vi "断电保存全局变量.vi"() -> ()   [LabVIEW 2016, in "环境动力监测库.lvlib"]
uses:
  <vilib>/Plasmionique/MB Master/MB_Master/MB_Master.lvclass
panel:
  in  "选项卡控件":T1(tab)
  in  "空调全局":T2={"型号选择"=enum."黑盾", "MB session in"=refnum, "英维克空调寄存器"=[], "通讯状态"=TRUE, "PORT"="502", "IP"="192.168.1.207", "Slave ID "=1, "Serial Config"={"baud rate (bps)"=9600, "stop bits"=10, "parity"=0, "flow control"=0, "timeout"=1000, "retries"=1}, "VISA Resource"="COM1", "MB通信方式选择"=enum."串口"} {"Serial Config"."stop bits" items=["1.0"=10, "1.5"=15, "2.0"=20]; "Serial Config"."flow control" items=["None", "XON/XOFF", "RTS/CTS", "XON/XOFF & RTS/CTS", "DTR/DSR", "XON/XOFF & DTR/DSR"]; "Serial Config"."parity" items=["None", "Odd", "Even", "Mark", "Space"]}
  in  "UPS全局":T3={"VISA resource name"="", "Serial Config"={"baud rate (9600)"=2400, "stop bits (10: 1 bit)"=10, "parity (0:none)"=enum."None", "data bits (8)"=8, "timeout (10sec)"=10000}, "型号选择"=enum."山特UPSC1~3", "HW-UPS-2000 MB session"=refnum, "连接方式"=enum."串口", "IP"="", "Port"=""} {"Serial Config"."data bits (8)" min=5 max=8 step=1; "Serial Config"."stop bits (10: 1 bit)" items=["1.0"=10, "1.5"=15, "2.0"=20]}
  out "累计用电量KW·h":dbl
  in  "MPPT-12 Serial":refnum<visa-resource-name>
  in  "MPPT-24 Serial":refnum<visa-resource-name>
  in  "MPPT12电量告警":dbl
  in  "MPPT24电量告警":dbl
  in  "MPPT-12Serial Config":T4={"baud rate (bps)"=115200, "stop bits"=10, "parity"=0, "flow control"=0, "timeout"=1000, "retries"=1} {"stop bits" items=["1.0"=10, "1.5"=15, "2.0"=20]; "parity" items=["None", "Odd", "Even", "Mark", "Space"]; "flow control" items=["None", "XON/XOFF", "RTS/CTS", "XON/XOFF & RTS/CTS", "DTR/DSR", "XON/XOFF & DTR/DSR"]}
  in  "MPPT-24Serial Config":T4={"baud rate (bps)"=115200, "stop bits"=10, "parity"=0, "flow control"=0, "timeout"=1000, "retries"=1} {"stop bits" items=["1.0"=10, "1.5"=15, "2.0"=20]; "parity" items=["None", "Odd", "Even", "Mark", "Space"]; "flow control" items=["None", "XON/XOFF", "RTS/CTS", "XON/XOFF & RTS/CTS", "DTR/DSR", "XON/XOFF & DTR/DSR"]}
  in  "MPPT-12站号":u64
  in  "MPPT-24站号":u64
  in  "纬度":dbl
  in  "经度":dbl
  in  "BD连接方式":enum16{"串口", "TCP"}(ring)
  in  "BDPort:":string
  in  "BDIP address:":string
  in  "GPS连接方式":enum16{"串口", "TCP"}(ring)
  in  "GPSPort:":string
  in  "GPSIP address:":string
  in  "手动设置定位":bool caption="定位自动获取OFF/手动设置ON"
  in  "收方地址":string="968314"
  in  "GPS移位报警设定值":dbl=1000.0
  in  "BD移位报警设定值":dbl=1000.0
  in  "GPS波特率":u32(ring)=115200 items=["4800"=4800, "9600"=9600, "38400"=38400, "19200"=19200, "115200"=115200]
  in  "GPS VISA资源名称":refnum<visa-resource-name>
  in  "BD波特率":u32(ring)=115200 items=["4800"=4800, "9600"=9600, "38400"=38400, "19200"=19200, "115200"=115200]
  in  "BDVISA资源名称":refnum<visa-resource-name>
  in  "室温上限告警点":dbl
  in  "室温下限告警点":dbl
  in  "湿度上限告警点":dbl
  in  "湿度下限告警点":dbl
  in  "高温告警开关":bool
  in  "冰箱参数":cluster{"功能启用":bool, "开启时间":u16, "关闭时间":u16}={"功能启用"=FALSE, "开启时间"=6, "关闭时间"=20} {"关闭时间" items=["00H", "01H", "02H", "03H", "04H", "05H", "06H", "07H", "08H", "09H", "10H", "11H", "12H", "13H", "14H", "15H", "16H", "17H", "18H", "19H", "20H", "21H", "22H", "23H", "关闭"]; "开启时间" items=["00H", "01H", "02H", "03H", "04H", "05H", "06H", "07H", "08H", "09H", "10H", "11H", "12H", "13H", "14H", "15H", "16H", "17H", "18H", "19H", "20H", "21H", "22H", "23H", "关闭"]}
  in  "排气扇参数":T5={"功能启用"=FALSE, "排气扇开启温度"=50.0, "排气扇关闭温度"=40.0}
  out "AD当前转换值":T6 {"AD7" format="%.2f"; "AD6" format="%.2f"; "AD5" format="%.2f"; "AD4" format="%.2f"; "AD3" format="%.2f"; "AD2" format="%.2f"; "AD1" format="%.2f"; "AD0" format="%.2f"}
  out "AD当前原始值":T7 {"AD7" format="%.2f"; "AD6" format="%.2f"; "AD5" format="%.2f"; "AD4" format="%.2f"; "AD3" format="%.2f"; "AD1" format="%.2f"; "AD1" format="%.2f"; "AD0" format="%.2f"}
  in  "AD线性关系":T8(array[cluster])=[{"X0"=1638.0, "X1"=8191.0, "Y0"=-40.0, "Y1"=100.0}, {"X0"=1638.0, "X1"=8191.0, "Y0"=0.0, "Y1"=100.0}, {"X0"=1638.0, "X1"=8191.0, "Y0"=0.0, "Y1"=1.0}, {"X0"=0.0, "X1"=8191.0, "Y0"=0.0, "Y1"=8191.0}, {"X0"=0.0, "X1"=8191.0, "Y0"=0.0, "Y1"=8191.0}, {"X0"=0.0, "X1"=8191.0, "Y0"=0.0, "Y1"=8191.0}, {"X0"=0.0, "X1"=8191.0, "Y0"=0.0, "Y1"=8191.0}, {"X0"=0.0, "X1"=8191.0, "Y0"=0.0, "Y1"=8191.0}]
  out "配置ItemNames":string[][](array[string])
  out "监测设备配置":T9
  in  "IO监测配置输入":T10
  in  "卡号信息":string[][](array[string])
  in  "红外入侵信号持续时间":u32=1 format="%.0fS"
  in  "漏水信号持续时间":u32=1 format="%.0fS"
  in  "门禁信号持续时间":u32=1 format="%.0fS"
  in  "烟雾信号持续时间":u32=1 format="%.0fS"
  in  "用水量信号持续时间":u32=1 format="%.0fS"
  in  "振动信号持续时间":u32=1 format="%.0fS"
  in  "废液信号持续时间":u32=1 format="%.0fS"
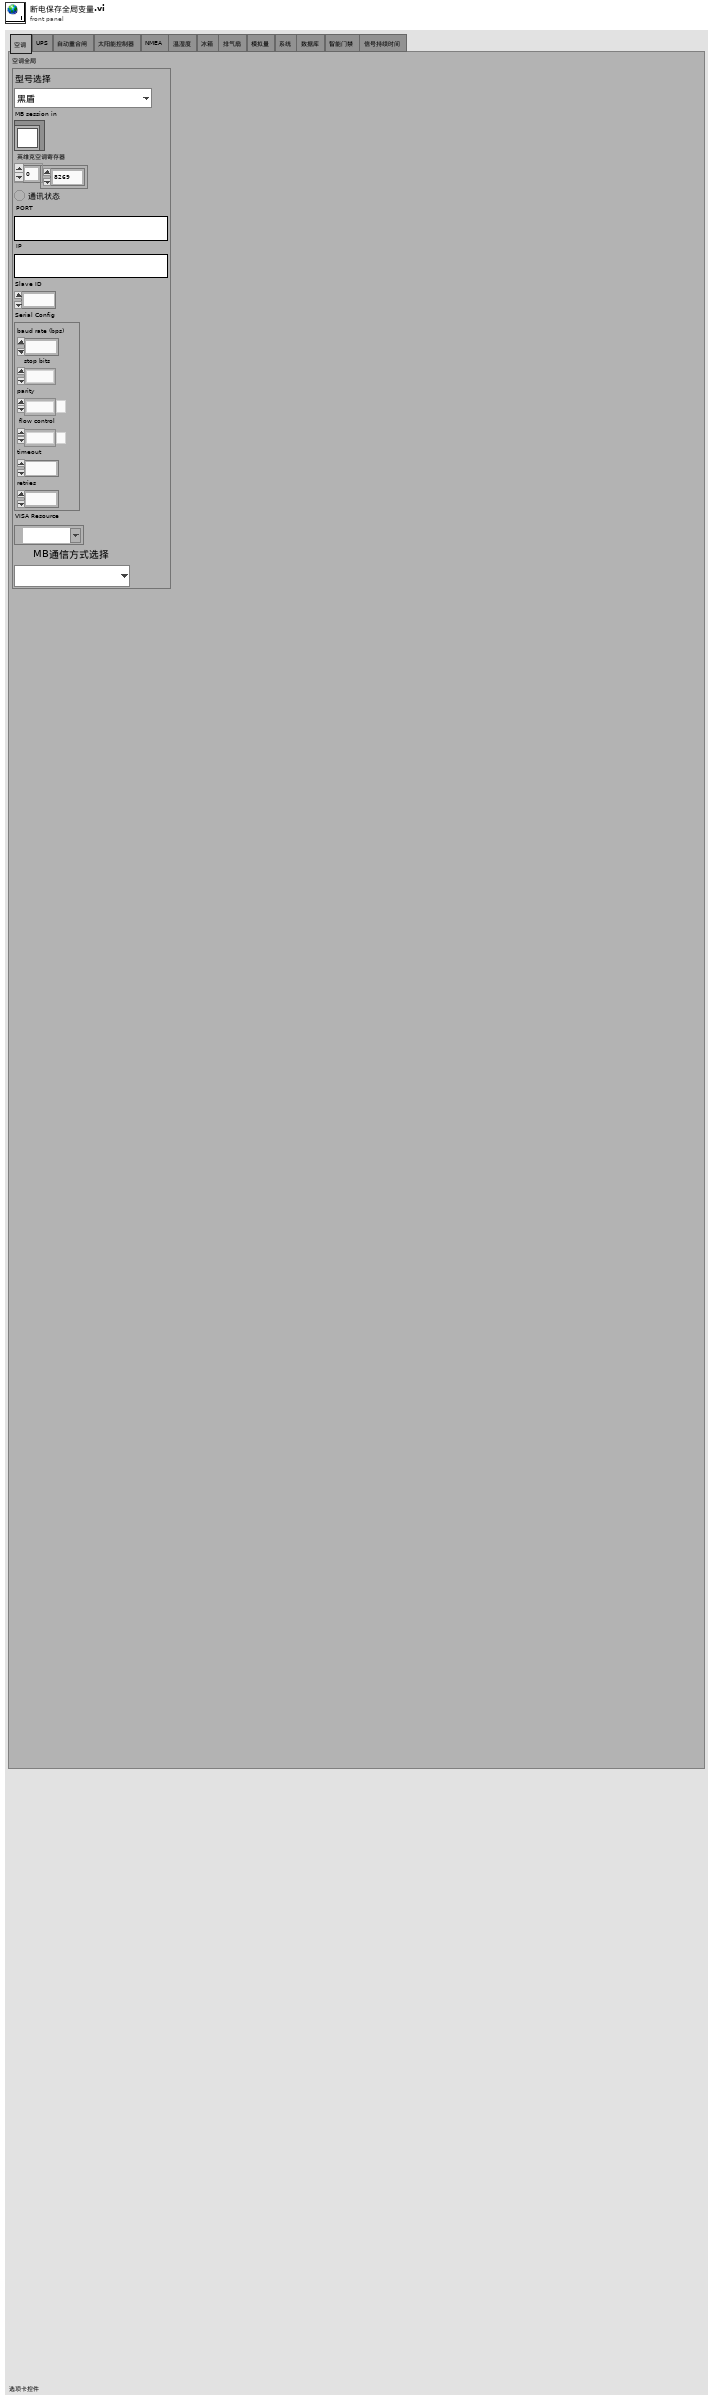
[diagram p1: front panel]
types:
  T1 = enum32{"空调", "UPS", "自动重合闸", "太阳能控制器", "NMEA", "温湿度", "冰箱", "排气扇", "模拟量", "系统", "数据库", "智能门禁", "信号持续时间"}
  T2 = cluster{"型号选择":enum16{"黑盾", "英维克", "仁科测控RS-KTC-N01"}, "MB session in":refnum<class "MB_Master.lvclass">, "英维克空调寄存器":u16[], "通讯状态":bool, "PORT":string, "IP":string, "Slave ID ":u8, "Serial Config":cluster{"baud rate (bps)":u32, "stop bits":u16, "parity":u16, "flow control":u16, "timeout":u32, "retries":i32}, "VISA Resource":refnum<visa-resource-name>, "MB通信方式选择":enum16{"串口", "TCP"}}
  T3 = cluster{"VISA resource name":refnum<visa-resource-name>, "Serial Config":cluster{"baud rate (9600)":u32, "stop bits (10: 1 bit)":u16, "parity (0:none)":enum16{"None", "Odd", "Even", "Mark", "Space"}, "data bits (8)":u16, "timeout (10sec)":u32}, "型号选择":enum16{"山特UPSC1~3", "山特UPSC6~20", "华为UPS2000-G-(1-3KVA)"}, "HW-UPS-2000 MB session":refnum<class "MB_Master.lvclass">, "连接方式":enum16{"串口", "TCP"}, "IP":string, "Port":string}
  T4 = cluster{"baud rate (bps)":u32, "stop bits":u16, "parity":u16, "flow control":u16, "timeout":u32, "retries":i32}
  T5 = cluster{"功能启用":bool, "排气扇开启温度":dbl, "排气扇关闭温度":dbl}
  T6 = cluster{"AD0":dbl, "AD1":dbl, "AD2":dbl, "AD3":dbl, "AD4":dbl, "AD5":dbl, "AD6":dbl, "AD7":dbl}
  T7 = cluster{"AD0":dbl, "AD1":dbl, "AD1":dbl, "AD3":dbl, "AD4":dbl, "AD5":dbl, "AD6":dbl, "AD7":dbl}
  T8 = cluster{"X0":dbl, "X1":dbl, "Y0":dbl, "Y1":dbl}[]
  T9 = cluster{"市电监测":bool, "用水量监测":bool, "烟雾监测":bool, "温度湿度":bool, "振动监测":bool, "红外入侵监测":bool, "漏水监测":bool, "门禁开关监测":bool, "门禁开关监测2":bool, "视频监测":bool, "UPS监测":bool, "空调监测":bool, "冰箱监测":bool, "排气扇监测":bool, "蓄电池监测":bool, "蓄电池监测2":bool, "GPS监测":bool, "北斗监测":bool, "气象监测":bool, "智能门禁监测":bool, "废液监测":bool, "废液监测2":bool}
  T10 = cluster{"漏水监测配置":cluster{"监测项描述:输出":string, "端口:":enum16{"AI0", "AI1", "AI2", "AI3", "AI4", "DI0", "DI1", "DI2", "DI3", "DI4", "DI5", "DI6", "DI7", "DO0", "DO1", "DO2", "DO3", "DO4", "DO5", "DO6", "DO7", "X0", "X1", "X2", "X3", "X4", "X5", "X6", "X7", "X8", "X9", "X10", "X11", "X12", "X13", "X14", "X15", "X16", "X17", "X18", "X19", "X20", "X21", "X22", "X23"}, "告警参数:":enum32{"禁用告警", "闭合告警", "断开告警"}, "传感器型号:":enum16{"PLC", "ZLAN", "ART"}, "声光告警启用":bool}, "门禁开关监测配置":cluster{"监测项描述:输出":string, "端口:":enum16{"AI0", "AI1", "AI2", "AI3", "AI4", "DI0", "DI1", "DI2", "DI3", "DI4", "DI5", "DI6", "DI7", "DO0", "DO1", "DO2", "DO3", "DO4", "DO5", "DO6", "DO7", "X0", "X1", "X2", "X3", "X4", "X5", "X6", "X7", "X8", "X9", "X10", "X11", "X12", "X13", "X14", "X15", "X16", "X17", "X18", "X19", "X20", "X21", "X22", "X23"}, "告警参数:":enum32{"禁用告警", "闭合告警", "断开告警"}, "传感器型号:":enum16{"PLC", "ZLAN", "ART"}, "声光告警启用":bool}, "门禁开关监测配置2":cluster{"监测项描述:输出":string, "端口:":enum16{"AI0", "AI1", "AI2", "AI3", "AI4", "DI0", "DI1", "DI2", "DI3", "DI4", "DI5", "DI6", "DI7", "DO0", "DO1", "DO2", "DO3", "DO4", "DO5", "DO6", "DO7", "X0", "X1", "X2", "X3", "X4", "X5", "X6", "X7", "X8", "X9", "X10", "X11", "X12", "X13", "X14", "X15", "X16", "X17", "X18", "X19", "X20", "X21", "X22", "X23"}, "告警参数:":enum32{"禁用告警", "闭合告警", "断开告警"}, "传感器型号:":enum16{"PLC", "ZLAN", "ART"}, "声光告警启用":bool}, "温湿度监测配置":cluster{"监测项描述:输出":string, "端口:":enum16{"AI0", "AI1", "AI2", "AI3", "AI4", "DI0", "DI1", "DI2", "DI3", "DI4", "DI5", "DI6", "DI7", "DO0", "DO1", "DO2", "DO3", "DO4", "DO5", "DO6", "DO7", "X0", "X1", "X2", "X3", "X4", "X5", "X6", "X7", "X8", "X9", "X10", "X11", "X12", "X13", "X14", "X15", "X16", "X17", "X18", "X19", "X20", "X21", "X22", "X23"}, "告警参数:":enum32{"禁用告警", "闭合告警", "断开告警"}, "传感器型号:":enum16{"PLC", "ZLAN", "ART"}, "声光告警启用":bool}, "烟雾监测配置":cluster{"监测项描述:输出":string, "端口:":enum16{"AI0", "AI1", "AI2", "AI3", "AI4", "DI0", "DI1", "DI2", "DI3", "DI4", "DI5", "DI6", "DI7", "DO0", "DO1", "DO2", "DO3", "DO4", "DO5", "DO6", "DO7", "X0", "X1", "X2", "X3", "X4", "X5", "X6", "X7", "X8", "X9", "X10", "X11", "X12", "X13", "X14", "X15", "X16", "X17", "X18", "X19", "X20", "X21", "X22", "X23"}, "告警参数:":enum32{"禁用告警", "闭合告警", "断开告警"}, "传感器型号:":enum16{"PLC", "ZLAN", "ART"}, "声光告警启用":bool}, "冰箱监测配置":cluster{"监测项描述:输出":string, "端口:":enum16{"AI0", "AI1", "AI2", "AI3", "AI4", "DI0", "DI1", "DI2", "DI3", "DI4", "DI5", "DI6", "DI7", "DO0", "DO1", "DO2", "DO3", "DO4", "DO5", "DO6", "DO7", "X0", "X1", "X2", "X3", "X4", "X5", "X6", "X7", "X8", "X9", "X10", "X11", "X12", "X13", "X14", "X15", "X16", "X17", "X18", "X19", "X20", "X21", "X22", "X23"}, "告警参数:":enum32{"禁用告警", "闭合告警", "断开告警"}, "传感器型号:":enum16{"PLC", "ZLAN", "ART"}, "声光告警启用":bool}, "排气扇监测配置":cluster{"监测项描述:输出":string, "端口:":enum16{"AI0", "AI1", "AI2", "AI3", "AI4", "DI0", "DI1", "DI2", "DI3", "DI4", "DI5", "DI6", "DI7", "DO0", "DO1", "DO2", "DO3", "DO4", "DO5", "DO6", "DO7", "X0", "X1", "X2", "X3", "X4", "X5", "X6", "X7", "X8", "X9", "X10", "X11", "X12", "X13", "X14", "X15", "X16", "X17", "X18", "X19", "X20", "X21", "X22", "X23"}, "告警参数:":enum32{"禁用告警", "闭合告警", "断开告警"}, "传感器型号:":enum16{"PLC", "ZLAN", "ART"}, "声光告警启用":bool}, "红外入侵监测配置":cluster{"监测项描述:输出":string, "端口:":enum16{"AI0", "AI1", "AI2", "AI3", "AI4", "DI0", "DI1", "DI2", "DI3", "DI4", "DI5", "DI6", "DI7", "DO0", "DO1", "DO2", "DO3", "DO4", "DO5", "DO6", "DO7", "X0", "X1", "X2", "X3", "X4", "X5", "X6", "X7", "X8", "X9", "X10", "X11", "X12", "X13", "X14", "X15", "X16", "X17", "X18", "X19", "X20", "X21", "X22", "X23"}, "告警参数:":enum32{"禁用告警", "闭合告警", "断开告警"}, "传感器型号:":enum16{"PLC", "ZLAN", "ART"}, "声光告警启用":bool}, "振动监测配置":cluster{"监测项描述:输出":string, "端口:":enum16{"AI0", "AI1", "AI2", "AI3", "AI4", "DI0", "DI1", "DI2", "DI3", "DI4", "DI5", "DI6", "DI7", "DO0", "DO1", "DO2", "DO3", "DO4", "DO5", "DO6", "DO7", "X0", "X1", "X2", "X3", "X4", "X5", "X6", "X7", "X8", "X9", "X10", "X11", "X12", "X13", "X14", "X15", "X16", "X17", "X18", "X19", "X20", "X21", "X22", "X23"}, "告警参数:":enum32{"禁用告警", "闭合告警", "断开告警"}, "传感器型号:":enum16{"PLC", "ZLAN", "ART"}, "声光告警启用":bool}, "废液监测配置":cluster{"监测项描述:输出":string, "端口:":enum16{"AI0", "AI1", "AI2", "AI3", "AI4", "DI0", "DI1", "DI2", "DI3", "DI4", "DI5", "DI6", "DI7", "DO0", "DO1", "DO2", "DO3", "DO4", "DO5", "DO6", "DO7", "X0", "X1", "X2", "X3", "X4", "X5", "X6", "X7", "X8", "X9", "X10", "X11", "X12", "X13", "X14", "X15", "X16", "X17", "X18", "X19", "X20", "X21", "X22", "X23"}, "告警参数:":enum32{"禁用告警", "闭合告警", "断开告警"}, "传感器型号:":enum16{"PLC", "ZLAN", "ART"}, "声光告警启用":bool}, "废液监测配置2":cluster{"监测项描述:输出":string, "端口:":enum16{"AI0", "AI1", "AI2", "AI3", "AI4", "DI0", "DI1", "DI2", "DI3", "DI4", "DI5", "DI6", "DI7", "DO0", "DO1", "DO2", "DO3", "DO4", "DO5", "DO6", "DO7", "X0", "X1", "X2", "X3", "X4", "X5", "X6", "X7", "X8", "X9", "X10", "X11", "X12", "X13", "X14", "X15", "X16", "X17", "X18", "X19", "X20", "X21", "X22", "X23"}, "告警参数:":enum32{"禁用告警", "闭合告警", "断开告警"}, "传感器型号:":enum16{"PLC", "ZLAN", "ART"}, "声光告警启用":bool}}
diagram:
